vi "Get Value at Pin - PAE.vi"(10 "Target Pin (dBm)":dbl, 11 "Measurement":dbl[][](array[numeric])) -> (3 "Value(s) at Pin":dbl[](array[numeric]))   [LabVIEW 2023]
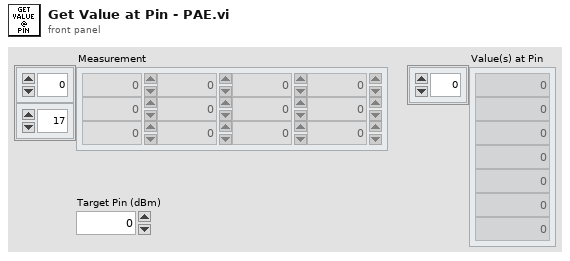
[diagram p1: front panel]
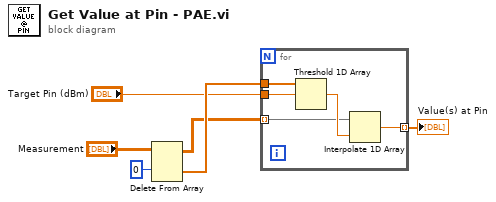
[diagram p0: block diagram]
diagram:
  n1 = Delete From Array(array="Measurement", index (row)=0) -> (deleted portion=w5:dbl[], array with subset deleted=w4:dbl[][])  [unwired: 2 in]
  n2 = for {
    tunnel: w4 -> [w7] mode=indexing
    tunnel: "Target Pin (dBm)" -> [w9]
    tunnel: w5 -> [w10]
    tunnel: [w11] -> w1 mode=indexing
    n3 = Threshold 1D Array(2:w9, 3:w10) -> (0:w8:dbl)  [unwired: 1 in]
    n4 = Interpolate 1D Array(1:w8, 2:w7) -> (0:w11:dbl)
  }
  "Value(s) at Pin" <- w1
